vi "mod_Generic Symbol Map Demonstration.vi"(0 "Generic Symbol Map Params":T1={"symbol values"=[[1, 17, 21, 5, 4, 20, 16, 0], [33, 49, 53, 37, 36, 52, 48, 32], [41, 57, 61, 45, 44, 60, 56, 40], [9, 25, 29, 13, 12, 28, 24, 8], [11, 27, 31, 15, 14, 30, 26, 10], [43, 59, 63, 47, 46, 62, 58, 42], [35, 51, 55, 39, 38, 54, 50, 34], [3, 19, 23, 7, 6, 22, 18, 2]], "symbol amplitudes (I)"=[-10.0, -8.0, -6.0, -4.0, 4.0, 6.0, 8.0, 10.0], "symbol amplitudes (Q)"=[10.0, 8.0, 6.0, 4.0, -4.0, -6.0, -8.0, -10.0], "gain"=108.0}, 11 "error in (no error)":errorcluster) -> (4 "symbol map":cdb[](array[numeric]), 15 "error out":errorcluster)   [LabVIEW 2020, in "niDMT.lvlib"]
uses:
  <vilib>/addons/Modulation/niDMT.lvlib
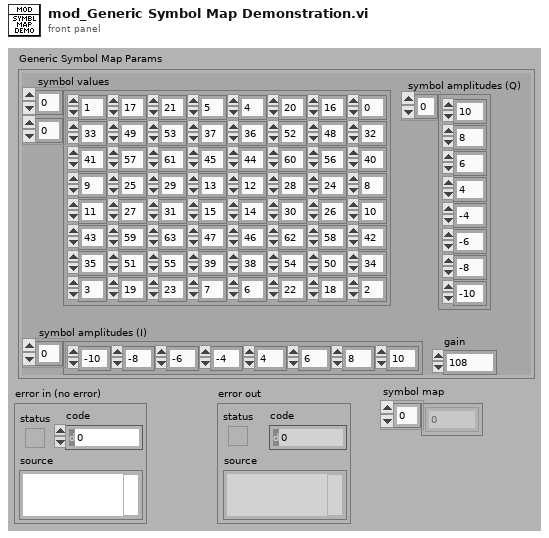
[diagram p1: front panel]
types:
  T1 = cluster{"symbol values":i32[][], "symbol amplitudes (I)":dbl[], "symbol amplitudes (Q)":dbl[], "gain":dbl}
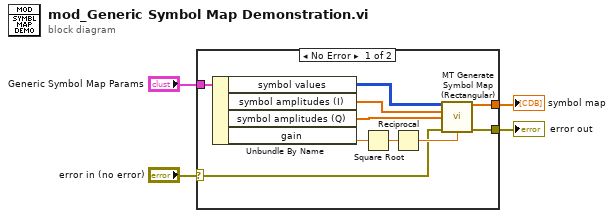
[diagram p0: block diagram]
diagram:
  n1 = case shown="No Error" "error in (no error)" {
    selector: "error in (no error)" -> [w6 w15]
    tunnel: [w14 _] -> w4
    tunnel: [w13 w15] -> w2
    tunnel: "Generic Symbol Map Params" -> [w7 _]
    frame No Error {
      n2 = Unbundle By Name(w7) -> ("symbol values"=w8:i32[][], "symbol amplitudes (I)"=w10:dbl[], "symbol amplitudes (Q)"=w9:dbl[], "gain"=w5:dbl)
      n3 = Square Root(x=w5) -> (sqrt(x)=w12:dbl)
      n4 = Reciprocal(x=w12) -> (1/x=w11:dbl)
      n5 = call <vilib>:"MT Generate Symbol Map (Rectangular).vi"("symbol values"=w8, "symbol amplitudes (I)"=w10, "symbol amplitudes (Q)"=w9, "error in (no error)"=w6, "gain"=w11) -> ("symbol map"=w14:cdb[], "error out"=w13:errorcluster)  [unwired: 9 out]
    }
    frame Error {
    }
  }
  "symbol map" <- w4
  "error out" <- w2
